vi "条件格式范围.vi"(5 "条件合适序号":i32=1, 7 "工作表名称":string="Sheet1", 8 "错误输入（无错误）":errorcluster, 11 "单元格区域":T1={"起始列"="A", "起始行"=1, "大小"=[]} {"大小" min=1 max=1048576; "起始行" min=1 max=1048576}) -> (0 "错误输出":errorcluster)   [LabVIEW 2020, in "OperateExcel.lvlib"]
uses:
  OperateExcel.lvlib
  Globals.vi
  <vilib>/Utility/error.llb/Error Cluster From Error Code.vi
  <vilib>/ErrorRing/Error Ring.xnode
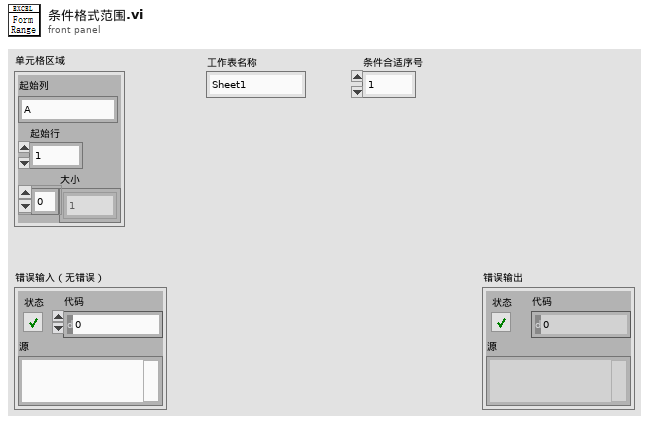
[diagram p1: front panel]
types:
  T1 = typedef "OperateExcel.lvlib/单元格区域.ctl" = cluster{"起始列":string, "起始行":u32, "大小":u32[]}
  T2 = typedef "OperateExcel.lvlib/引用簇.ctl" = cluster{"Excel._Application":refnum<k7>, "Workbooks":refnum<k7>, "Open":refnum<k7>, "Worksheets":refnum<k7>, "sheetList":refnum<k7>[]}
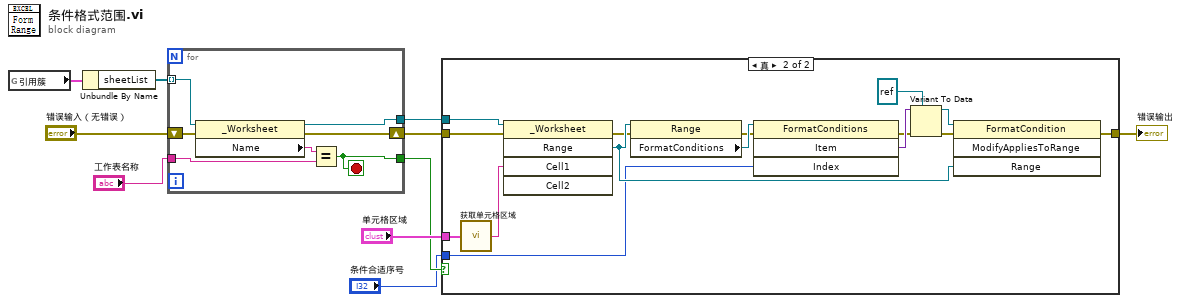
[diagram p0: block diagram]
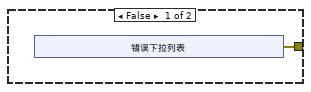
[diagram p2: hidden frame]
diagram:
  n1 = global read "Globals.vi" "引用簇"() -> (w3:T2)
  n2 = Unbundle By Name(w3) -> ("sheetList"=w10:refnum<k7>[])
  n3 = for {
    tunnel: w10 -> [w17] mode=indexing
    tunnel: "工作表名称" -> [w15]
    tunnel: [w14] -> w9
    shift-right: [w12] -> w7
    shift-left: "错误输入（无错误）" -> [w13]
    tunnel: [w11] -> w2
    stop <- w11 stop-if-true
    n4 = property class="_Worksheet"(reference=w17, error in=w13) -> (reference out=w14:refnum<k7>, error out=w12:errorcluster, "Name"=w16:string)
    n5 = Equal?(x=w16, y=w15) -> (x = y?=w11:bool)
  }
  n6 = case shown="真" w2 {
    tunnel: w9 -> [_ w37]
    tunnel: w7 -> [_ w36]
    tunnel: [w18 w24] -> w6
    tunnel: "单元格区域" -> [_ w35]
    tunnel: "条件合适序号" -> [_ w23]
    frame False {
      n7 = xnode "错误下拉列表"() -> ("错误输出"=w18:errorcluster)
    }
    frame True {
      n8 = call "获取单元格区域.vi"("单元格区域"=w35) -> ("单元格区域"=w32:string)
      n9 = invoke class="_Worksheet" method="Range"(reference=w37, error in=w36, "Cell1"=w32) -> (error out=w28:errorcluster, "Range"=w29:refnum<k7>)  [unwired: 2 in, 3 out]
      n10 = property class="Range"(reference=w29, error in=w28) -> (error out=w27:errorcluster, "FormatConditions"=w31:refnum<k7>)  [unwired: 1 out]
      n11 = invoke class="FormatConditions" method="Item"(reference=w31, error in=w27, "Index"=w23) -> (error out=w26:errorcluster, "Item"=w34:variant)  [unwired: 1 in, 2 out]
      n12 = Variant To Data(error in=w26, type=refnum<k7> refnum ("引用输出"), Variant=w34) -> (data=w30:refnum<k7>, error out=w25:errorcluster)
      n13 = invoke class="FormatCondition" method="ModifyAppliesToRange"(reference=w30, error in=w25, "Range"=w29) -> (error out=w24:errorcluster)  [unwired: 1 in, 3 out]
    }
  }
  "错误输出" <- w6
